vi "Read Response.vi"(6 "Timeout (ms)":i32=5000, 8 "error in (no error)":errorcluster, 10 "Number of Elements":u32, 11 "FPGA Interface in":refnum<class "FPGA Interface.lvclass">) -> (0 "error out":errorcluster, 2 "Data":u64[](array[numeric]), 4 "Elements Remaining":u32)   [LabVIEW 2020, in "BCI-1553 API.lvlib" / "FPGA Interface.lvlib" / "FPGA Interface.lvclass"]
doc: "Reads response data from the specified component in the 1553 Session."
uses:
  FPGA Interface.lvclass
  FPGA Interface.lvclass/FPGA Interface.ctl
  <vilib>/Utility/error.llb/Error Cluster From Error Code.vi
  <vilib>/rvi/errors/niLvFpgaAdjustHostInterfaceError.vi
  <vilib>/rvi/interface/nirviMethod/nirviMethod.xnode
  <vilib>/FPGAPlugInAG/Dynamic/niLvFpga_ReadFifo_Dynamic.vi
  <vilib>/rvi/errors/niLvFpgaMergeErrorWithErrorCode.vi
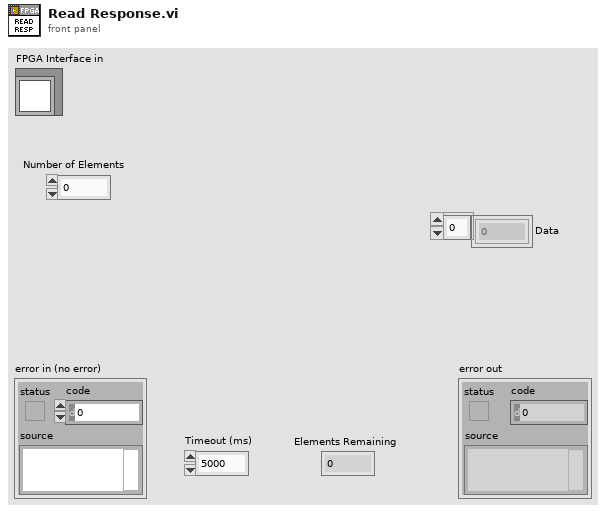
[diagram p1: front panel]
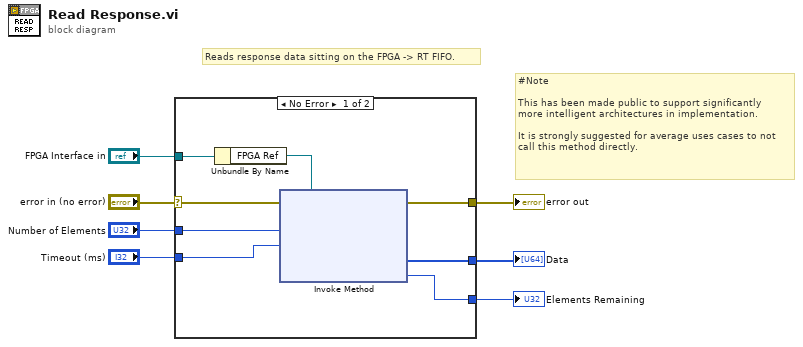
[diagram p0: block diagram]
diagram:
  # "#Note\n\nThis has been made public to support significantly\nmore intelligent architectures in implementation.\n\nIt is strongly suggested for average uses cases to not\ncall this method directly."
  # "Reads response data sitting on the FPGA -> RT FIFO."
  n1 = case shown="No Error" "error in (no error)" {
    selector: "error in (no error)" -> [w13 w16]
    tunnel: [w12 w16] -> w6
    tunnel: "FPGA Interface in" -> [w15 _]
    tunnel: "Number of Elements" -> [w11 _]
    tunnel: "Timeout (ms)" -> [w10 _]
    tunnel: [w9 _] -> w2
    tunnel: [w8 _] -> w1
    frame No Error {
      n2 = Unbundle By Name(w15) -> ("FPGA Ref"=w14:refnum<k20>)
      n3 = xnode "Invoke Method"("FPGA VI Reference In"=w14, "error in"=w13, "Number of Elements"=w11, "Timeout (ms)"=w10) -> ("error out"=w12:errorcluster, "Data"=w9:u64[], "Elements Remaining"=w8:u32)  [unwired: 1 out]
    }
    frame Error {
    }
  }
  "error out" <- w6
  "Data" <- w2
  "Elements Remaining" <- w1
